vi "Sim Config(Session&Bearer).vi"(8 "error constant":errorcluster, 11 "Session_array":T1(array[cluster])) -> (0 "error constant":errorcluster, 3 "Session_array 2":T1(array[cluster]))   [LabVIEW 2021]
uses:
  APIs/Controls/Base_Station_Emulator.ctl
  IP Simulation/Controls/Enum-TypeDef.ctl
panel:
  in  "Close":bool
  in  "Add Session":bool
  in  "Enum":T2
  in  "Base Station":T3
  # "Sessions & Bearers"
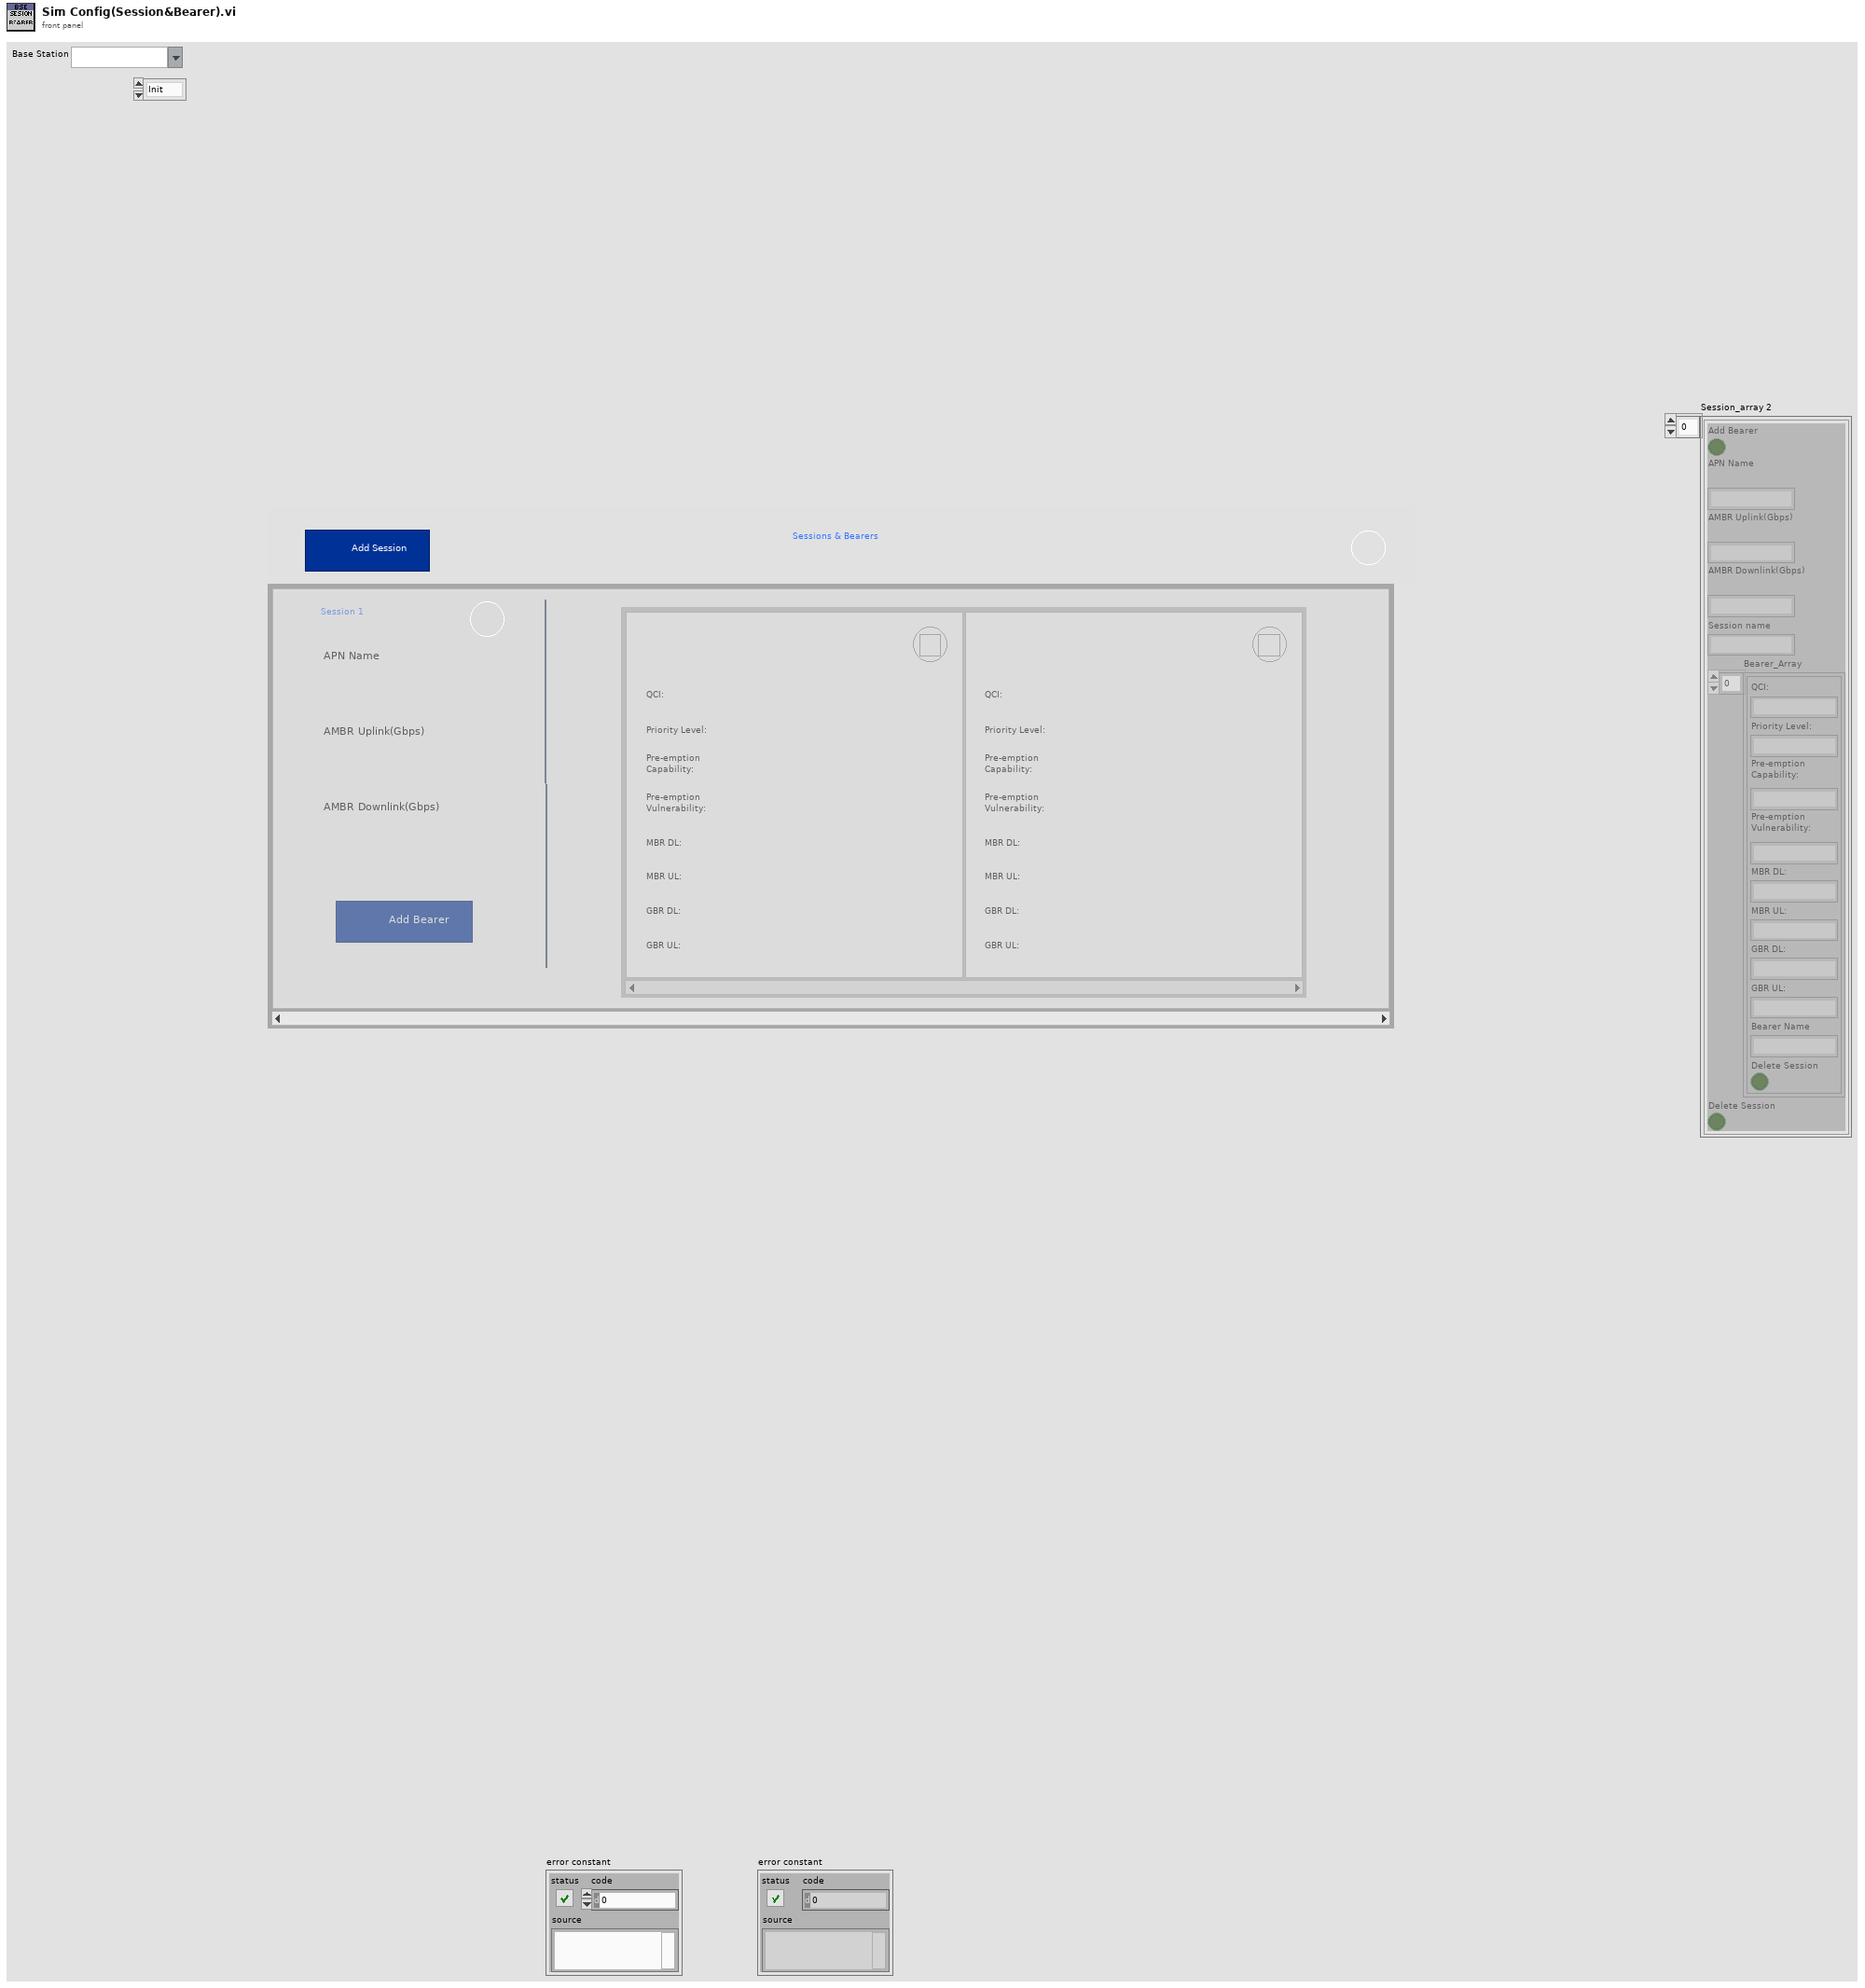
[diagram p1: front panel]
types:
  T1 = cluster{"Add Bearer":bool, "APN Name\n":string, "AMBR Uplink(Gbps)\n":string, "AMBR Downlink(Gbps)\n":string, "Session name":string, "Bearer_Array":cluster{"QCI:":string, "Priority Level:":string, "Pre-emption\nCapability:":string, "Pre-emption\nVulnerability:":string, "MBR DL:":string, "MBR UL:":string, "GBR DL:":string, "GBR UL:":string, "Bearer Name":string, "Delete Session":bool}[], "Delete Session":bool}[]
  T2 = typedef "Enum-TypeDef.ctl" = enum16{"Init", "poll", "Close"}
  T3 = typedef "Base_Station_Emulator.ctl" = string
  T4 = cluster{"Session_array":cluster{"Delete Session":bool, "Session name":string, "AMBR Downlink(Gbps)\n":string, "AMBR Uplink(Gbps)\n":string, "APN Name\n":string, "Add Bearer":bool}[], "Session & Bearer":cluster{"Bearer_Array":cluster{"QCI:":string, "Priority Level:":string, "Pre-emption\nCapability:":string, "Pre-emption\nVulnerability:":string, "MBR DL:":string, "MBR UL:":string, "GBR DL:":string, "GBR UL:":string, "Bearer Name":string, "Delete Session":bool}[], "Delete Session":bool}}
  T5 = cluster{"Add Bearer":bool, "APN Name\n":string, "AMBR Uplink(Gbps)\n":string, "AMBR Downlink(Gbps)\n":string, "Session name":string, "Bearer_Array":cluster{"QCI:":string, "Priority Level:":string, "Pre-emption\nCapability:":string, "Pre-emption\nVulnerability:":string, "MBR DL:":string, "MBR UL:":string, "GBR DL:":string, "GBR UL:":string, "Bearer Name":string, "Delete Session":bool}[], "Delete Session":bool}
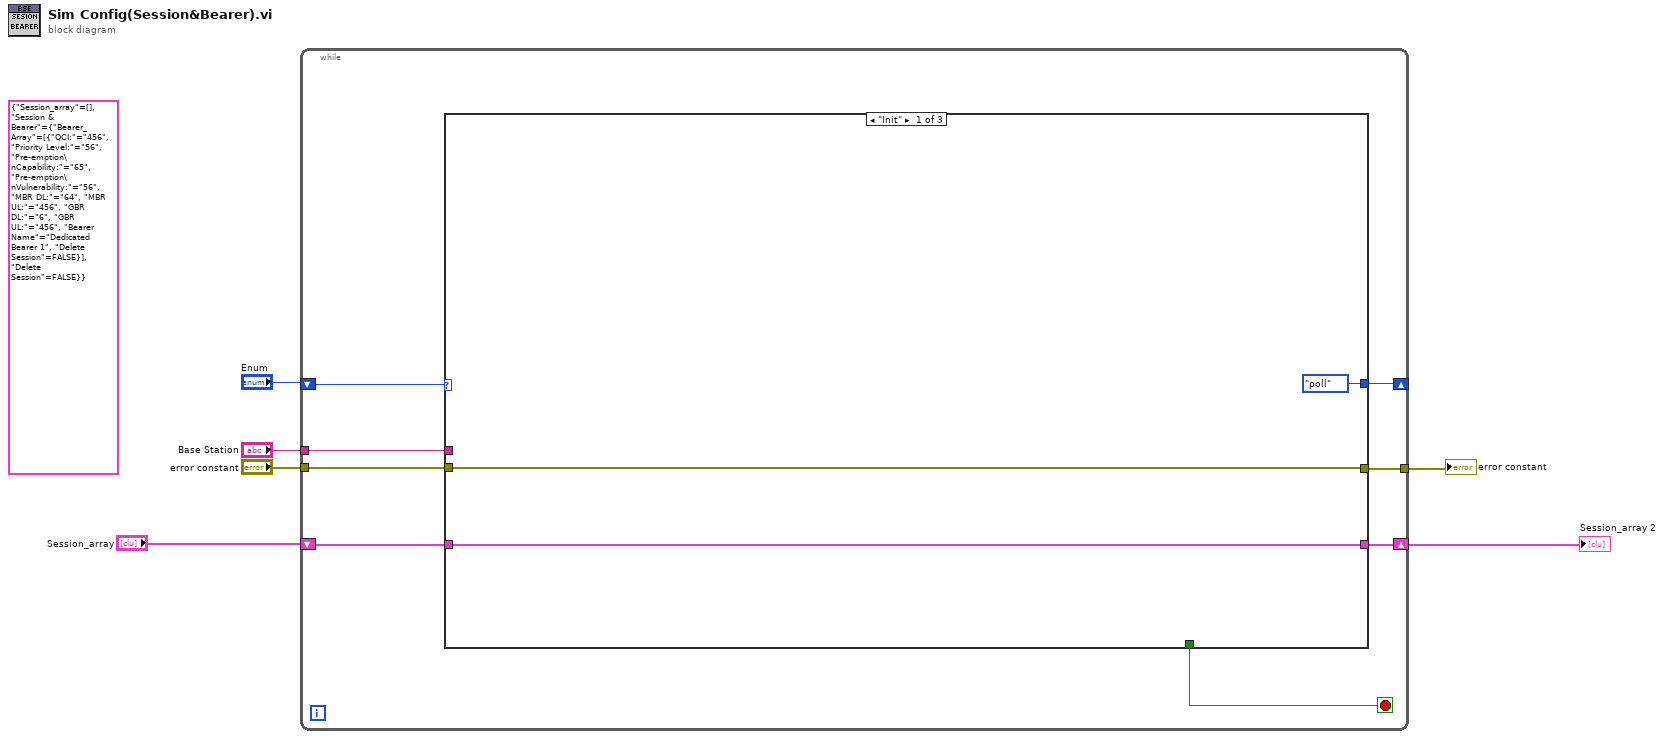
[diagram p0: block diagram]
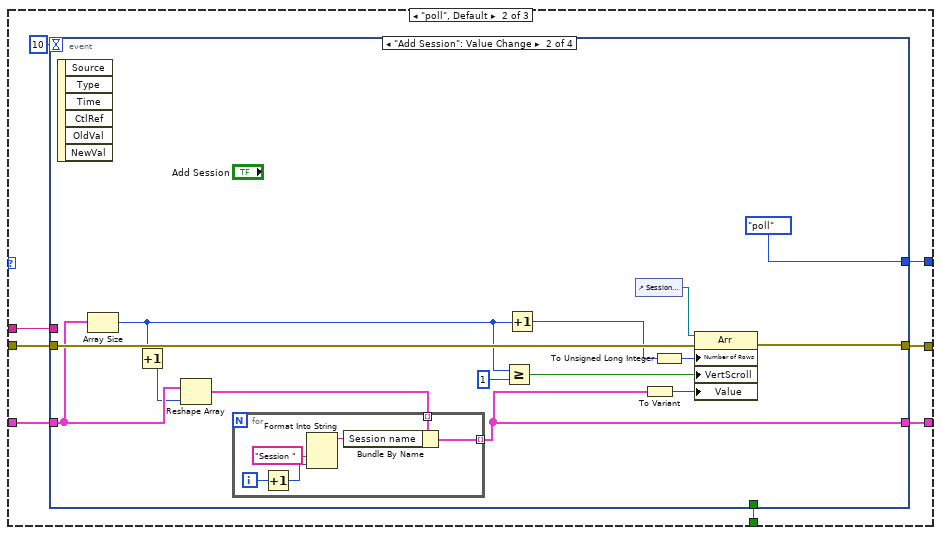
[diagram p2: hidden frame]
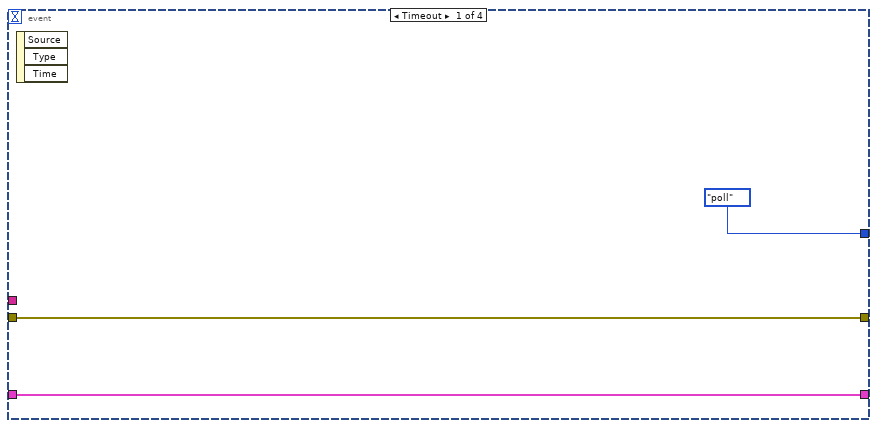
[diagram p3: hidden frame]
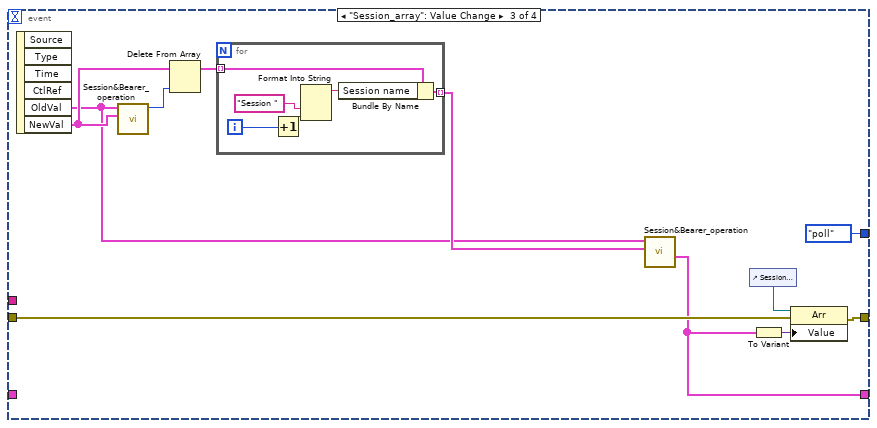
[diagram p4: hidden frame]
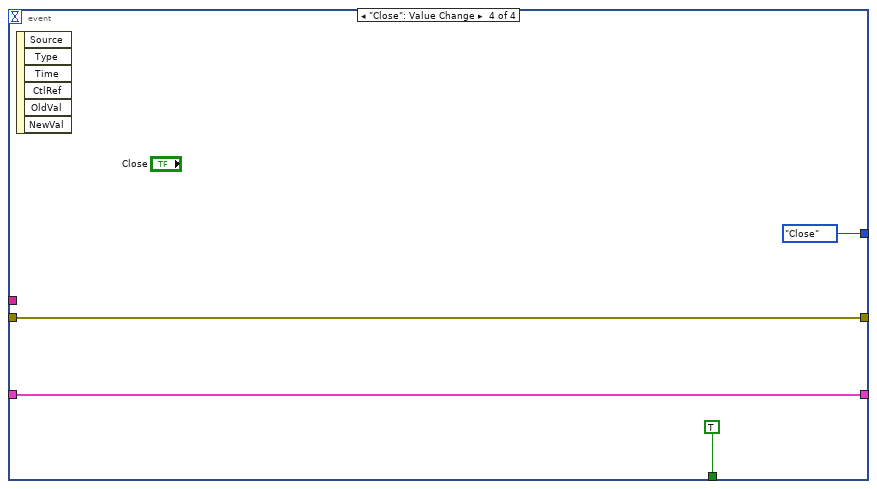
[diagram p5: hidden frame]
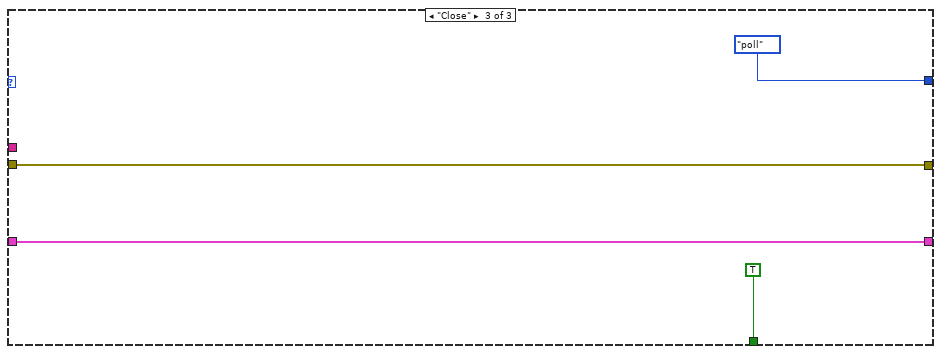
[diagram p6: hidden frame]
diagram:
  (unwired) T4 {"Session_array"=[], "Session & Bearer"={"Bearer_Array"=[{"QCI:"="456", "Priority Level:"="56", "Pre-emption\nCapability:"="65", "Pre-emption\nVulnerability:"="56", "MBR DL:"="64", "MBR UL:"="456", "GBR DL:"="6", "GBR UL:"="456", "Bearer Name"="Dedicated Bearer 1", "Delete Session"=FALSE}], "Delete Session"=FALSE}}
  n1 = while {
    shift-right: [w12] -> _
    shift-left: "Enum" -> [w13]
    tunnel: "error constant" -> [w11]
    tunnel: [w10] -> w3
    tunnel: "Base Station" -> [w9]
    shift-right: [w7] -> w1
    shift-left: "Session_array" -> [w8]
    stop <- w14 stop-if-true
    n2 = case shown="\"Init\"" w13 {
      tunnel: [_ w20 TRUE] -> w14
      tunnel: [Enum-TypeDef."poll" w23 Enum-TypeDef."poll"] -> w12
      tunnel: w11 -> [w16 w25 w72]
      tunnel: [w16 w24 w72] -> w10
      tunnel: w9 -> [_ w21 _]
      tunnel: w8 -> [w15 w19 w70]
      tunnel: [w15 w18 w70] -> w7
      frame "Init" {
      }
      frame "poll", Default {
        n3 = event shown="[1] \"Add Session\": Value Change" {
          selector: _ -> [_ _ _ _]
          dyn-events: _ -> [_ _ _ _]
          timeout: 10 -> [_ _ _ _]
          tunnel: w25 -> [w27 w38 w55 w68]
          tunnel: [w27 w39 w53 w68] -> w24
          tunnel: [Enum-TypeDef."poll" Enum-TypeDef."poll" Enum-TypeDef."poll" Enum-TypeDef."Close"] -> w23
          tunnel: w21 -> [_ _ _ _]
          tunnel: [_ _ _ TRUE] -> w20
          tunnel: w19 -> [w26 w33 _ w66]
          tunnel: [w26 w29 w52 w66] -> w18
          event Timeout {
            n4 = event-data() -> ()  [unwired: 1 in, 3 out]
          }
          event "Add Session": Value Change {
            n5 = event-data() -> ()  [unwired: 1 in, 6 out]
            n6 = Array Size(array=w33) -> (size(s)=w32:i32)
            n7 = Increment(x=w32) -> (x+1=w31:i32)
            n8 = Reshape Array(w33, w31) -> (w30:T1)
            n9 = for {
              tunnel: [w46] -> w29 mode=indexing
              tunnel: w30 -> [w45] mode=indexing
              i -> [w44]
              n10 = Increment(x=w44) -> (x+1=w43:i32)
              n11 = Format Into String("Session " ("resulting string"), w43) -> (resulting string=w47:string)  [unwired: 3 in, 1 out]
              n12 = Bundle By Name(cluster=w45, "Session name"=w47) -> (w46:T5)
            }
            n13 = Greater Or Equal?(x=w32, y=1) -> (x >= y?=w40:bool)
            n14 = Increment(x=w32) -> (x+1=w34:i32)
            n15 = control-ref of="Session_array"() -> (w37:refnum<vi>)
            n16 = To Variant(anything=w29) -> (Variant=w36:variant)
            n17 = To Unsigned Long Integer(number=w34) -> (unsigned 32bit integer=w35:u32)
            n18 = property class="Arr"(reference=w37, error in=w38, "Number of Rows"=w35, "VertScroll"=w40, "Value"=w36) -> (error out=w39:errorcluster)  [unwired: 1 out]
          }
          event "Session_array": Value Change {
            n19 = event-data() -> ("OldVal"=w49:T1, "NewVal"=w57:T1)  [unwired: 1 in, 4 out]
            n20 = call "Session&Bearer_operation.vi"("NewVal"=w57, "OldVal"=w49) -> ("Delete Index"=w58:i32)  [unwired: 7 in, 2 out]
            n21 = Delete From Array(array=w57, index=w58) -> (array with subset deleted=w50:T1)  [unwired: 1 in, 1 out]
            n22 = for {
              tunnel: w50 -> [w65] mode=indexing
              tunnel: [w64] -> w51 mode=indexing
              i -> [w61]
              n23 = Increment(x=w61) -> (x+1=w60:i32)
              n24 = Format Into String("Session " ("resulting string"), w60) -> (resulting string=w63:string)  [unwired: 3 in, 1 out]
              n25 = Bundle By Name(cluster=w65, "Session name"=w63) -> (w64:T5)
            }
            n26 = call "Session&Bearer_operation.vi"("NewVal"=w51, "OldVal"=w49) -> ("output array"=w52:T1)  [unwired: 7 in, 2 out]
            n27 = control-ref of="Session_array"() -> (w56:refnum<vi>)
            n28 = To Variant(anything=w52) -> (Variant=w54:variant)
            n29 = property class="Arr"(reference=w56, error in=w55, "Value"=w54) -> (error out=w53:errorcluster)  [unwired: 1 out]
          }
          event "Close": Value Change {
            n30 = event-data() -> ()  [unwired: 1 in, 6 out]
          }
        }
      }
      frame "Close" {
      }
    }
  }
  "error constant" <- w3
  "Session_array 2" <- w1
